vi "数据查询.vi"() -> ()   [LabVIEW 2016]
uses:
  <vilib>/Utility/sysdir.llb/System Directory Type.ctl
  <vilib>/Utility/miscctls.llb/LVPointTypeDef.ctl
panel:
  in  "数据查询菜单":enum32{"数据查询", "仪器数据", "操作日志", "报警信息", "调试数据"}(xcontrol)
  out "Error to Convert":i32(ring)=56 items=["无错误", "参数错误", "内存已满", "超出区域", "文件结束", "文件已打开", "一般文件IO错误", "未找到文件", "文件权限错误", "磁盘已满", "路径副本", "打开过多文件", "未启用", "未找到资源文件", "无法添加资源", "未找到资源", "未找到图像", "图像内存错误", "画笔不存在", "配置错误类型", "配置未找到解析段", "配置解析错误", "配置内存错误", "错误外部代码格式", "错误外部代码偏移量", "外部代码不存在", "空窗口", "销毁窗口错误", "空菜单", "打印已中止", "错误打印记录", "打印驱动程序错误", "打印时窗口错误", "打印时内存错误", "打印对话框错误", "一般打印错误", "无效设备引用句柄", "设备未找到", "设备参数错误", "设备单位错误", "无法打开设备", "设备调用已中止", "一般错误", "用户已取消", "对象ID过低", "对象ID过高", "对象不在堆中", "未知的堆", "错误DefProc ID", "DefProc不在表格中", "范围外信息", "空方法", "未知信息", "不支持管理器调用", "错误地址", "连接过程中", "连接超时", "连接过程中", "不支持网络属性", "网络错误", "正在使用的地址", "系统缺少内存", "连接已中止", "连接已拒绝", "连接未建立", "连接已建立", "连接已关闭", "初始化错误（交互应用程序管理器）", "错误事件发生", "等待无约束事件发生处理程序", "事件发生队列溢出", "错误路径", "未发出信号量", "未识别类型（交互应用程序管理器）"]
  in  "保存数据":bool
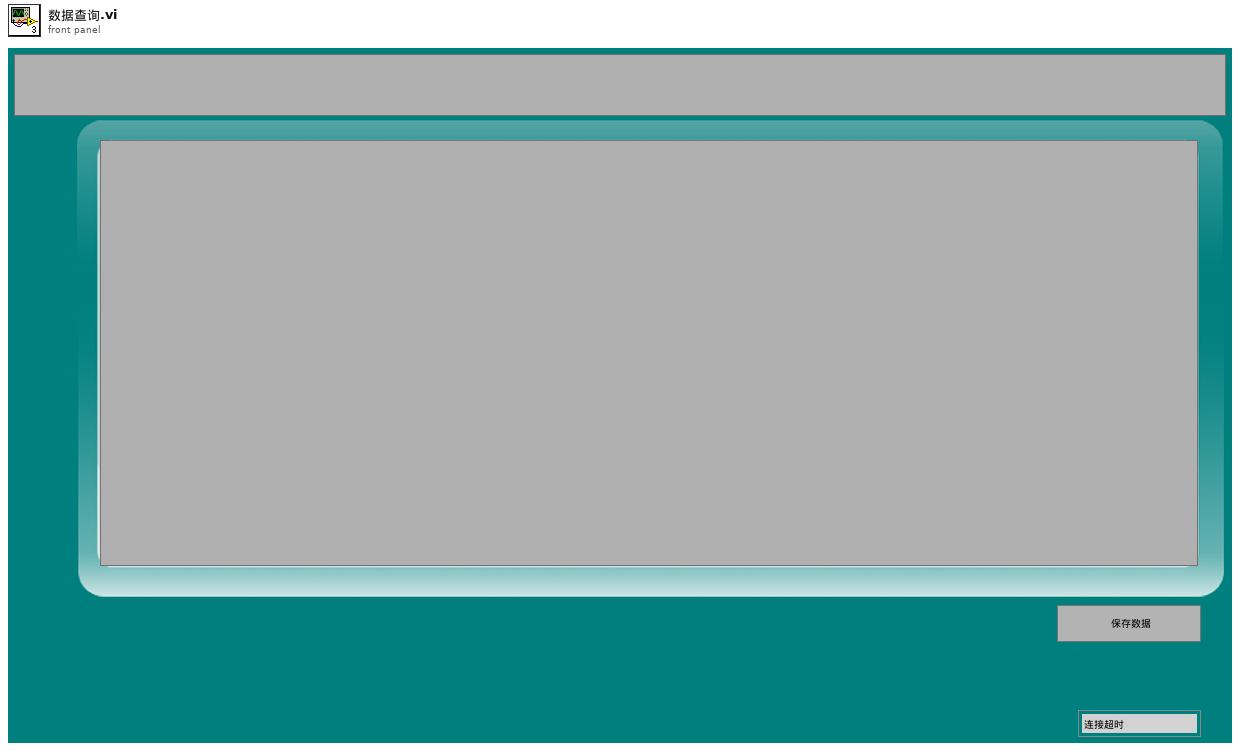
[diagram p1: front panel]
types:
  T1 = typedef "LVPointTypeDef.ctl" = cluster{"Horizontal":i16, "Vertical":i16}
  T2 = enum32{"Bad", "Idle", "Run top level", "Running"}
  T3 = typedef "System Directory Type.ctl" = i32
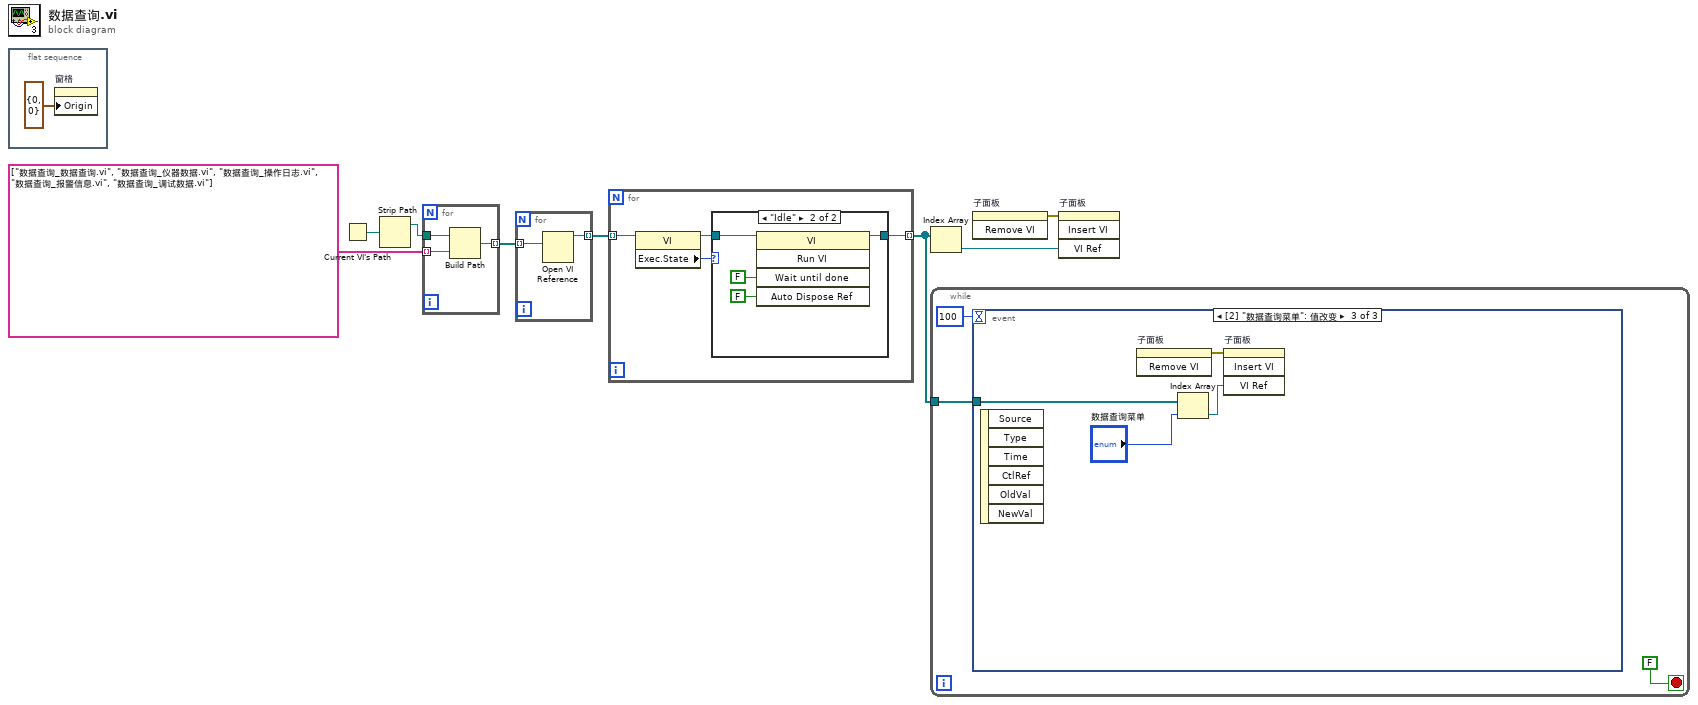
[diagram p0: block diagram]
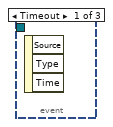
[diagram p3: hidden frame]
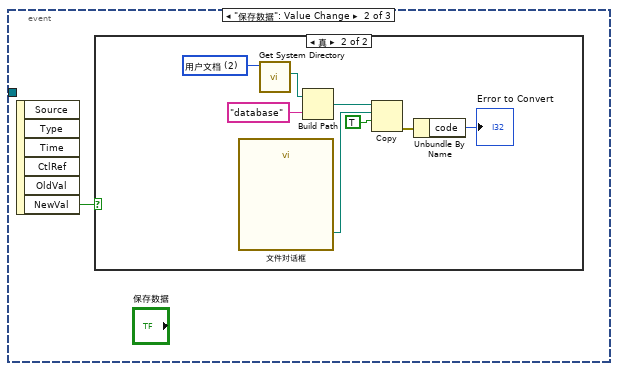
[diagram p4: hidden frame]
diagram:
  n1 = flat-sequence {
    frame #0 {
      n2 = property on="窗格" class="Pane"("Origin"=T1 {"Horizontal"=0, "Vertical"=0} ("原点")) -> ()  [unwired: 2 in, 2 out]
    }
  }
  n3 = Current VI's Path() -> (path=w8:path)
  n4 = Strip Path(path=w8) -> (stripped path=w7:path)  [unwired: 1 out]
  n5 = for {
    tunnel: w7 -> [w12]
    tunnel: string[] ["数据查询_数据查询.vi", "数据查询_仪器数据.vi", "数据查询_操作日志.vi", "数据查询_报警信息.vi", "数据查询_调试数据.vi"] -> [w11] mode=indexing
    tunnel: [w10] -> w5 mode=indexing
    n6 = Build Path(base path=w12, name or relative path=w11) -> (appended path=w10:path)
  }
  n7 = for {
    tunnel: w5 -> [w14] mode=indexing
    tunnel: [w13] -> w4 mode=indexing
    n8 = Open VI Reference(vi path=w14) -> (vi reference=w13:refnum<vi>)  [unwired: 5 in, 1 out]
  }
  n9 = for {
    tunnel: w4 -> [w18] mode=indexing
    tunnel: [w15] -> w2 mode=indexing
    n10 = property class="VI"(reference=w18) -> (reference out=w16:refnum<vi>, "Exec.State"=w17:T2)  [unwired: 1 in, 1 out]
    n11 = case shown="\"Idle\"" w17 {
      tunnel: w16 -> [w19 w21]
      tunnel: [w19 w20] -> w15
      frame "Bad", Default {
      }
      frame "Idle" {
        n12 = invoke class="VI" method="Run VI"(reference=w21, "Wait until done"=FALSE ("结束前等待"), "Auto Dispose Ref"=FALSE ("自动销毁引用")) -> (reference out=w20:refnum<vi>)  [unwired: 2 in, 4 out]
      }
    }
  }
  n13 = Index Array(array=w2) -> (element=w1:refnum<vi>)  [unwired: 1 in]
  n14 = while {
    tunnel: w2 -> [w25]
    stop <- FALSE stop-if-true
    n15 = event shown="[2] \"数据查询菜单\": 值改变" {
      selector: _ -> [_ _ _]
      dyn-events: _ -> [_ _ _]
      timeout: 100 -> [_ _ _]
      tunnel: w25 -> [_ _ w39]
      event Timeout {
        n16 = event-data() -> ()  [unwired: 1 in, 3 out]
      }
      event "保存数据": Value Change {
        n17 = event-data() -> ("NewVal"=w27:bool)  [unwired: 1 in, 5 out]
        n18 = case shown="真" w27 {
          frame False {
          }
          frame True {
            w35 = T3 2 items=["用户目录"=0, "用户桌面"=1, "用户文档"=2, "用户应用程序数据"=3, "用户设置"=4, "用户临时目录"=5, "公共文档"=6, "公共应用程序数据"=7, "公共设置"=8, "公共缓存"=13, "系统核心库"=9, "系统安装库"=10, "应用程序文件"=11, "启动盘根目录"=12] ("system directory type")
            n19 = call "文件对话框"() -> ("selected path"=w28:path)  [unwired: 12 in, 3 out]
            n20 = call <vilib>:"Get System Directory.vi"("system directory type"=w35) -> ("system directory"=w34:path)  [unwired: 10 in]
            n21 = Build Path(base path=w34, name or relative path="database" ("名称或相对路径")) -> (appended path=w32:path)
            n22 = Copy(9:TRUE ("覆盖(F)"), 10:w28, 11:w32) -> (0:w30:errorcluster)  [unwired: 2 in, 2 out]
            n23 = Unbundle By Name(w30) -> ("code"=→"Error to Convert":i32)
          }
        }
      }
      event "数据查询菜单": Value Change {
        n24 = event-data() -> ()  [unwired: 1 in, 6 out]
        n25 = invoke on="子面板" class="SubPnl" method="Remove VI"() -> (error out=w36:errorcluster)  [unwired: 3 in, 2 out]
        n26 = Index Array(array=w39, index="数据查询菜单") -> (element=w37:refnum<vi>)
        n27 = invoke on="子面板" class="SubPnl" method="Insert VI"(error in=w36, "VI Ref"=w37) -> ()  [unwired: 2 in, 4 out]
      }
    }
  }
  n28 = invoke on="子面板" class="SubPnl" method="Remove VI"() -> (error out=w3:errorcluster)  [unwired: 3 in, 2 out]
  n29 = invoke on="子面板" class="SubPnl" method="Insert VI"(error in=w3, "VI Ref"=w1) -> ()  [unwired: 2 in, 4 out]
